vi "排序.vi"(1 "数组":T1[](array[typedef])) -> (0 "已排序":T1[](array[typedef]))   [LabVIEW 2020]
uses:
  acd1ed76-f654-47b4-b16c-3f82427c7923.vi
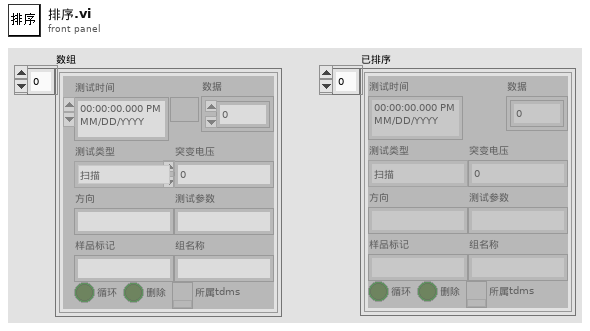
[diagram p1: front panel]
types:
  T1 = typedef "测试数据类型.ctl" = cluster{"测试时间":timestamp, "测试类型":T2, "方向":string, "样品标记":string, "测试参数":string, "循环":bool, "删除":bool, "组名称":string, "所属tdms":refnum<k34>, "突变电压":i32, "数据":dbl[][]}
  T2 = typedef "测试类型.ctl" = enum16{"扫描", "脉冲", "维持时间"}
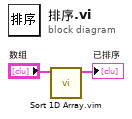
[diagram p0: block diagram]
diagram:
  n1 = call "Sort 1D Array.vim"("unsorted array"="数组") -> ("sorted array"=→"已排序":T1[])  [unwired: 10 in]
